vi "TCPFrameProc.vi"(11 "input arrray":u8[](array[numeric])) -> ()   [LabVIEW 2021]
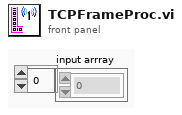
[diagram p1: front panel]
types:
  T1 = cluster{"Valve compensator HT":bool, "Valve compensator LT ":bool, "Temperature module HT":bool, "Temperature module LT":bool, "Pressure module":bool, "Power module":bool}
  T2 = cluster{"ValvePos1":sgl, "ValvePos2":sgl, "PressureArray":sgl[], "TempArray2":sgl[], "TempArray1":sgl[], "Time Stamp":timestamp}[]
  T3 = cluster{"ValvePos1":sgl, "ValvePos2":sgl, "PressureArray":sgl[], "TempArray2":sgl[], "TempArray1":sgl[], "Time Stamp":timestamp}
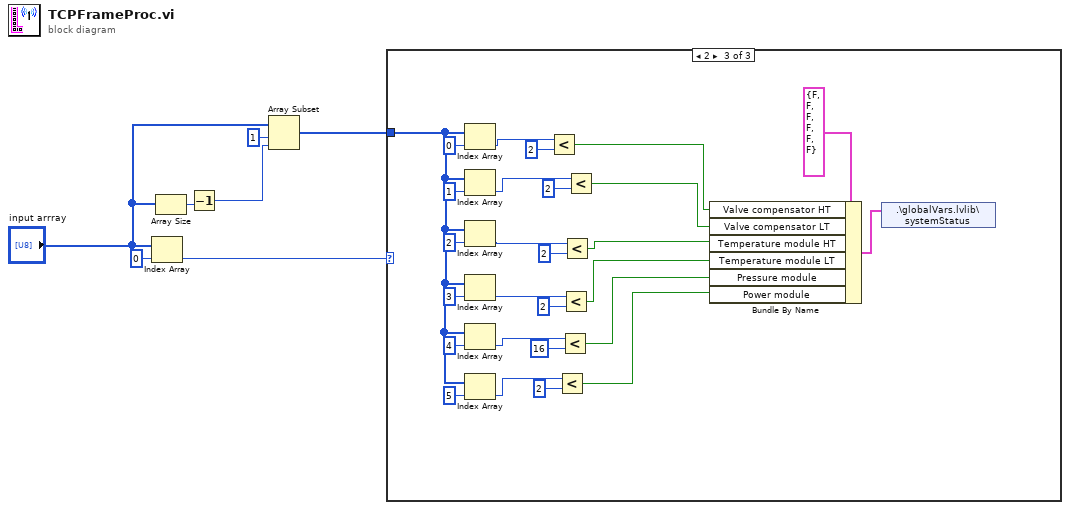
[diagram p0: block diagram]
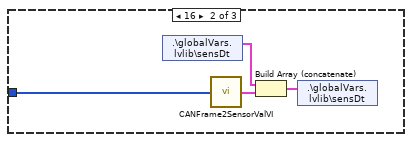
[diagram p3: hidden frame]
diagram:
  n1 = Index Array(array="input arrray", index=0) -> (element=w2:u8)
  n2 = Array Size(array="input arrray") -> (size(s)=w5:i32)
  n3 = Decrement(x=w5) -> (x-1=w6:i32)
  n4 = Array Subset(array="input arrray", index=1, length=w6) -> (w7:u8[])
  n5 = case shown="2" w2 {
    tunnel: w7 -> [_ w8 w38]
    frame 0, Default {
    }
    frame 16 {
      n6 = shared-variable ".\\globalVars.lvlib\\sensDt"() -> (w11:T2)  [unwired: 1 in, 1 out]
      n7 = call "CANFrame2SensorValVI.vi"("input"=w8) -> ("output cluster"=w10:T3)
      n8 = Build Array (concatenate)(w11, w10) -> (w9:T2)
      n9 = shared-variable ".\\globalVars.lvlib\\sensDt"(w9) -> ()  [unwired: 1 in, 1 out]
    }
    frame 2 {
      n10 = Index Array(array=w38, index=0) -> (element=w29:u8)
      n11 = Index Array(array=w38, index=1) -> (element=w17:u8)
      n12 = Index Array(array=w38, index=2) -> (element=w18:u8)
      n13 = Index Array(array=w38, index=3) -> (element=w19:u8)
      n14 = Index Array(array=w38, index=4) -> (element=w20:u8)
      n15 = Index Array(array=w38, index=5) -> (element=w21:u8)
      n16 = Less?(x=w29, y=u8 2) -> (x < y?=w27:bool)
      n17 = Less?(x=w21, y=u8 2) -> (x < y?=w12:bool)
      n18 = Less?(x=w20, y=u8 16) -> (x < y?=w13:bool)
      n19 = Less?(x=w19, y=u8 2) -> (x < y?=w14:bool)
      n20 = Less?(x=w18, y=u8 2) -> (x < y?=w15:bool)
      n21 = Less?(x=w17, y=u8 2) -> (x < y?=w16:bool)
      n22 = Bundle By Name(cluster=T1 {"Valve compensator HT"=FALSE, "Valve compensator LT "=FALSE, "Temperature module HT"=FALSE, "Temperature module LT"=FALSE, "Pressure module"=FALSE, "Power module"=FALSE} ("systemStatus"), "Valve compensator HT"=w27, "Valve compensator LT"=w16, "Temperature module HT"=w15, "Temperature module LT"=w14, "Pressure module"=w13, "Power module"=w12) -> (w30:T1)
      n23 = shared-variable ".\\globalVars.lvlib\\systemStatus"(w30) -> ()  [unwired: 1 in, 1 out]
    }
  }
